vi "String2Hex.vi"(1 "String":string) -> (0 "Hex":string)   [LabVIEW 2012]
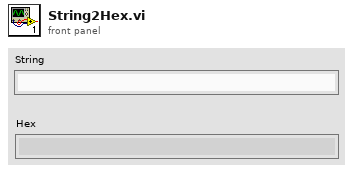
[diagram p1: front panel]
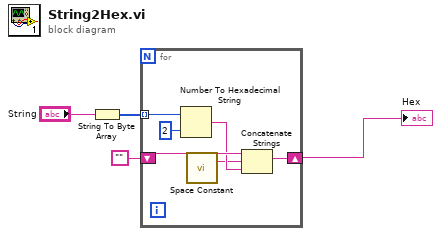
[diagram p0: block diagram]
diagram:
  n1 = String To Byte Array(string="String") -> (unsigned byte array=w3:u8[])
  n2 = for {
    tunnel: w3 -> [w10] mode=indexing
    shift-right: [w8] -> w2
    shift-left: "" -> [w7]
    n3 = Number To Hexadecimal String(1:i16 2 ("宽度(-)"), 2:w10) -> (0:w6:string)
    n4 = call <vilib>:"Space Constant.vi"() -> ("String"=w5:string)
    n5 = Concatenate Strings(w7, w5, w6) -> (w8:string)
  }
  "Hex" <- w2
